vi "process.memory.dump.vi"(11 "Memory.dump.in":u64[](array[numeric])=[43520, 11, 0, 0, 47872, 32, 0, 47873, 0, 0, 0, 0, 1, 0, 0, 0, 2, 0, 0, 0, 3, 0, 0, 0, 4, 0, 0, 0, 5, 0, 0, 0, 6, 0, 0, 0, 7, 0, 0, 0, 8, 0, 0, 0, 9, 0, 0, 0, 10, 49, 20000, 1, 11, 0, 0, 0, 12, 0, 0, 0, 13, 0, 0, 0, 14, 0, 0, 0, 15, 0, 0, 0, 16, 0, 0, 0, 17, 0, 0, 0, 18, 0, 0, 0, 19, 0, 0, 0, 20, 48, 20000, 1, 21, 0, 0, 0, 22, 0, 0, 0, 23, 0, 0, 0, 24, 0, 0, 0, 25, 0, 0, 0, 26, 0, 0, 0, 27, 0, 0, 0, 28, 0, 0, 0, 29, 0, 0, 0, 30, 0, 0, 0, 31, 0, 0, 0, 48128, 32, 1, 48129, 0, 0, 0, 0, 1, 0, 0, 0, 2, 0, 0, 0, 3, 0, 0, 0, 4, 0, 0, 0, 5, 0, 0, 0, 6, 0, 0, 0, 7, 51, 100, 1, 8, 0, 0, 0, 9, 0, 0, 0, 10, 0, 0, 0, 11, 0, 0, 0, 12, 0, 0, 0, 13, 0, 0, 0, 14, 0, 0, 0, 15, 0, 0, 0, 16, 0, 0, 0, 17, 0, 0, 0, 18, 0, 0, 0, 19, 0, 0, 0, 20, 0, 0, 0, 21, 0, 0, 0, 22, 0, 0, 0, 23, 0, 0, 0, 24, 0, 0, 0, 25, 0, 0, 0, 26, 0, 0, 0, 27, 0, 0, 0, 28, 0, 0, 0, 29, 0, 0, 0, 30, 0, 0, 0, 31, 0, 0, 0] format="%.0x") -> (2 "mem.bank.1":cluster{"address":i32, "order.slot.hm":T1}[](array[cluster])=[{"address"=7, "order.slot.hm"={"OrderId"=51, "Quantity"=100, "IsValid"=TRUE}}] {"order.slot.hm"."OrderId" format="%016x"}, 3 "mem.bank.0":cluster{"address":i32, "order.slot.hm":T1}[](array[cluster])=[{"address"=10, "order.slot.hm"={"OrderId"=49, "Quantity"=20000, "IsValid"=TRUE}}, {"address"=20, "order.slot.hm"={"OrderId"=48, "Quantity"=20000, "IsValid"=TRUE}}] {"address" format="%.0x"; "order.slot.hm"."OrderId" format="%016x"})   [LabVIEW 2020]
uses:
  fpga/order.slot.hm.ctl
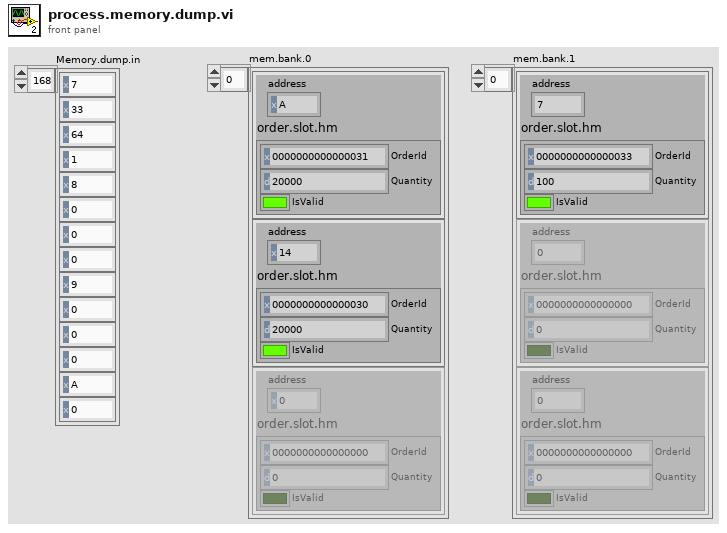
[diagram p1: front panel]
types:
  T1 = typedef "order.slot.hm.ctl" = cluster{"OrderId":u64, "Quantity":u64, "IsValid":bool}
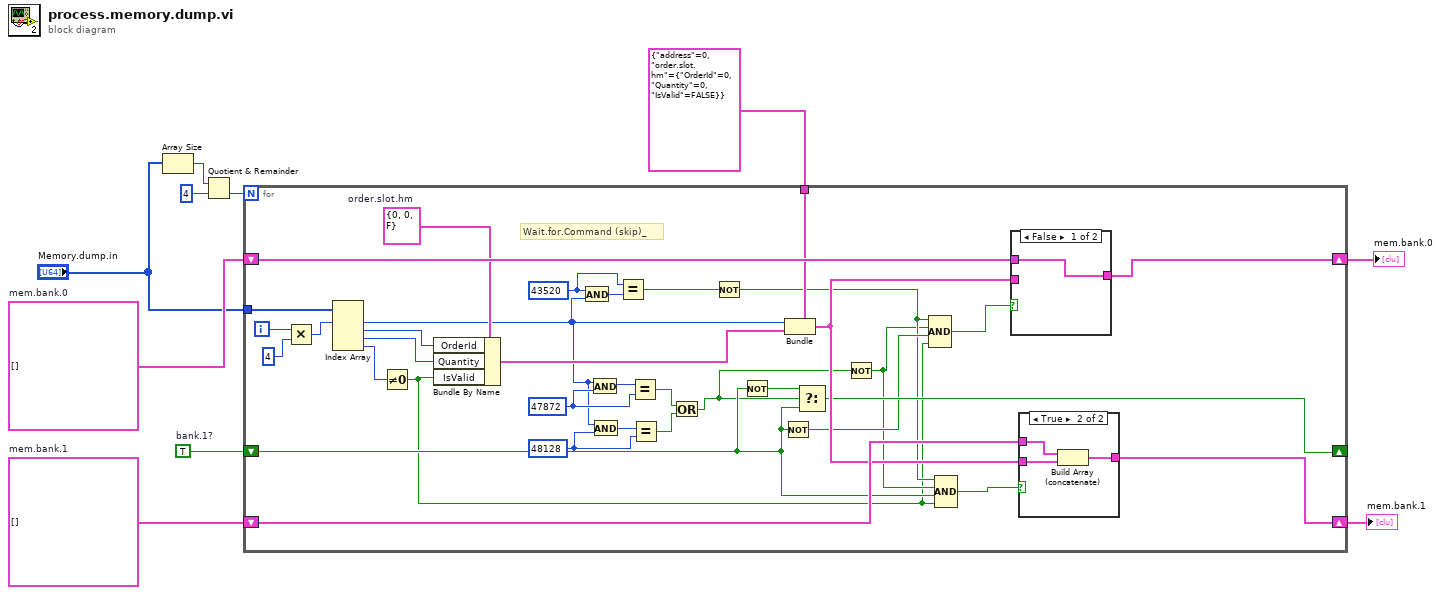
[diagram p0: block diagram]
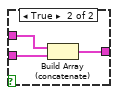
[diagram p3: hidden frame]
diagram:
  w2 = TRUE  # bank.1?
  w3 = cluster{"address":i32, "order.slot.hm":T1}[] []  # mem.bank.1
  w8 = cluster{"address":i32, "order.slot.hm":T1}[] []  # mem.bank.0
  n1 = Array Size(array="Memory.dump.in") -> (size(s)=w4:i32)
  n2 = Quotient & Remainder(x=w4, y=4) -> (floor(x/y)=w6:i32)  [unwired: 1 out]
  n3 = for {
    N: w6 -> [_]
    shift-right: [w40] -> w10
    shift-left: w8 -> [w41]
    tunnel: "Memory.dump.in" -> [w45]
    tunnel: cluster{"address":i32, "order.slot.hm":T1} {"address"=0, "order.slot.hm"={"OrderId"=0, "Quantity"=0, "IsValid"=FALSE}} -> [w38]
    shift-right: [w31] -> w1
    shift-left: w3 -> [w30]
    shift-right: [w23] -> _
    shift-left: w2 -> [w18]
    i -> [w44]
    w15 = u64 48128 ("x")
    w26 = u64 47872 ("x")
    w32 = u64 43520 ("x")
    w37 = T1 {"OrderId"=0, "Quantity"=0, "IsValid"=FALSE}  # order.slot.hm
    # "Wait.for.Command (skip)_"
    n4 = Multiply(x=w44, y=4) -> (x*y=w42:i32)
    n5 = Index Array(array=w45, index #1=w42) -> (element #1=w12:u64, element #2=w35:u64, element #3=w36:u64, element #4=w39:u64)  [unwired: 3 in]
    n6 = Not Equal To 0?(x=w39) -> (x != 0?=w17:bool)
    n7 = Bundle By Name(cluster=w37, "OrderId"=w35, "Quantity"=w36, "IsValid"=w17) -> (w34:T1)
    n8 = And(x=w32, y=w12) -> (x .and. y?=w33:u64)
    n9 = And(x=w12, y=w26) -> (x .and. y?=w25:u64)
    n10 = And(x=w12, y=w15) -> (x .and. y?=w14:u64)
    n11 = Equal?(x=w32, y=w33) -> (x = y?=w27:bool)
    n12 = Equal?(x=w25, y=w26) -> (x = y?=w16:bool)
    n13 = Equal?(x=w14, y=w15) -> (x = y?=w13:bool)
    n14 = Or(x=w16, y=w13) -> (x .or. y?=w11:bool)
    n15 = Not(x=w27) -> (.not. x?=w21:bool)
    n16 = Not(x=w18) -> (.not. x?=w24:bool)
    n17 = Not(x=w18) -> (.not. x?=w22:bool)
    n18 = Bundle(cluster=w38, "address"=w12, "order.slot.hm"=w34) -> (w29:cluster{"address":i32, "order.slot.hm":T1})
    n19 = Select(t=w24, s=w11, f=w18) -> (s? t:f=w23:bool)
    n20 = Not(x=w11) -> (.not. x?=w19:bool)
    n21 = Compound Arithmetic op=AND(w21, w19, w22, w17) -> (w28:bool)
    n22 = Compound Arithmetic op=AND(w21, w19, w18, w17) -> (w20:bool)
    n23 = case shown="False" w28 {
      tunnel: w41 -> [w50 w53]
      tunnel: [w50 w52] -> w40
      tunnel: w29 -> [_ w51]
      frame False {
      }
      frame True {
        n24 = Build Array (concatenate)(w53, w51) -> (w52:cluster{"address":i32, "order.slot.hm":T1}[])
      }
    }
    n25 = case shown="True" w20 {
      tunnel: w30 -> [w46 w49]
      tunnel: [w46 w48] -> w31
      tunnel: w29 -> [_ w47]
      frame False {
      }
      frame True {
        n26 = Build Array (concatenate)(w49, w47) -> (w48:cluster{"address":i32, "order.slot.hm":T1}[])
      }
    }
  }
  "mem.bank.0" <- w10
  "mem.bank.1" <- w1
